vi "Pre Launch Init.vi"(11 "MiniGUI in":refnum<class "MiniGUI.lvclass">) -> (0 "error out":errorcluster, 3 "MiniGUI out":refnum<class "MiniGUI.lvclass">)   [LabVIEW 2019, in "MiniGUI.lvlib" / "MiniGUI.lvclass"]
doc: "Initializes the panel actor. Creates the Panel Helper.\n\n----\nPlease see the following web address for additional documentation and tutorial information:\nhttp://www.mooregoodideas.com/mgi-panel-manager/\n\nAuthor: Derek Trepanier\n\nCopyright (c) 2018, Moore Good Ideas, Inc.\n\nAll rights reserved.\n\nRedistribution and use in source and binary forms, with or without modification, are permitted provided that the following conditions are met:\n\n * Redistributions of source code must retain the above copyright notice, this list of conditions and the following disclaimer.\n * Redistributions in binary form must reproduce the above copyright notice, this list of conditions and the following disclaimer in the documentation and/or other materials provided with the distribution.\n * Neither the name of Moore Good Ideas, Inc. nor the names of its contributors may be used to endorse or promote products derived from this software without specific prior written permission.\n\nTHIS SOFTWARE IS PROVIDED BY THE COPYRIGHT HOLDERS AND CONTRIBUTORS \"AS IS\" AND ANY EXPRESS OR IMPLIED WARRANTIES, INCLUDING, BUT NOT LIMITED TO, THE IMPLIED WARRANTIES OF MERCHANTABILITY AND FITNESS FOR A PARTICULAR PURPOSE ARE DISCLAIMED. IN NO EVENT SHALL THE COPYRIGHT OWNER OR CONTRIBUTORS BE LIABLE FOR ANY DIRECT, INDIRECT, INCIDENTAL, SPECIAL, EXEMPLARY, OR CONSEQUENTIAL DAMAGES (INCLUDING, BUT NOT LIMITED TO, PROCUREMENT OF SUBSTITUTE GOODS OR SERVICES; LOSS OF USE, DATA, OR PROFITS; OR BUSINESS INTERRUPTION) HOWEVER CAUSED AND ON ANY THEORY OF LIABILITY, WHETHER IN CONTRACT, STRICT LIABILITY, OR TORT (INCLUDING NEGLIGENCE OR OTHERWISE) ARISING IN ANY WAY OUT OF THE USE OF THIS SOFTWARE, EVEN IF ADVISED OF THE POSSIBILITY OF SUCH DAMAGE."
uses:
  MiniGUI.lvclass
  Dataset GUI.ctl
  LabGUI Head.ctl
  MiniGUI.lvclass/MiniGUI.ctl
  <vilib>/MGI/Panel Manager/Panel Actor/Panel Actor/Panel Actor.lvclass
  MiniGUI.lvlib
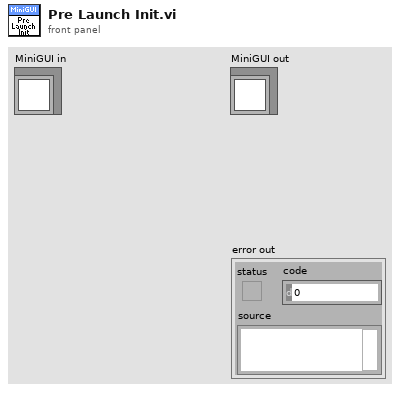
[diagram p1: front panel]
types:
  T1 = typedef "LabGUI Head.ctl" = cluster{"SV":dbl, "PV":dbl, "String":string, "Color Box":u32, "FeedBack":enum16{""}}
  T2 = cluster{"Compressor":bool, "M1":T1, "M2":T1, "Error":string, "System Name":string, "dual head":bool}
  T3 = typedef "MiniGUI.lvlib/Dataset GUI.ctl" = cluster{"M1 Status":cluster{"Read Temp":dbl[unit], "Bin String":string, "M1 Set Temp":dbl[unit], "Feedback":u8}, "M2 Status":cluster{"Read Temp":dbl[unit], "Bin String":string, "M2 Set Temp":dbl[unit], "Feedback":u8}}
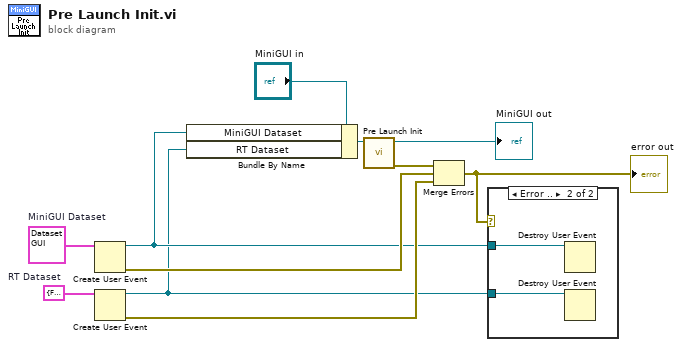
[diagram p0: block diagram]
diagram:
  w2 = T2 {"Compressor"=FALSE, "M1"={"SV"=0.0, "PV"=0.0, "String"="", "Color Box"=0, "FeedBack"=enum.""}, "M2"={"SV"=0.0, "PV"=0.0, "String"="", "Color Box"=0, "FeedBack"=enum.""}, "Error"="", "System Name"="", "dual head"=FALSE}  # RT Dataset
  w4 = T3 {"M1 Status"={"Read Temp"=393.25, "Bin String"="", "M1 Set Temp"=393.65, "Feedback"=1}, "M2 Status"={"Read Temp"=393.25, "Bin String"="", "M2 Set Temp"=393.65, "Feedback"=1}}  # MiniGUI Dataset
  n1 = Create User Event(user event datatype=w4) -> (user event=w3:refnum<user-event>, error out=w7:errorcluster)  [unwired: 1 in]
  n2 = Create User Event(user event datatype=w2) -> (user event=w1:refnum<user-event>, error out=w5:errorcluster)  [unwired: 1 in]
  n3 = Bundle By Name(cluster="MiniGUI in", "MiniGUI Dataset"=w3, "RT Dataset"=w1) -> (w6:refnum<class "MiniGUI.lvclass">)
  n4 = call-parent "Pre Launch Init.vi"("Panel Actor in"=w6) -> ("error out"=w10:errorcluster, "Panel Actor out"=→"MiniGUI out":refnum<class "MiniGUI.lvclass">)  [unwired: 9 in]
  n5 = Merge Errors(w10, w7, w5) -> (w9:errorcluster)
  "error out" <- w9
  n6 = case shown="Error .." w9 {
    tunnel: w3 -> [_ w13]
    tunnel: w1 -> [_ w12]
    frame No Error {
    }
    frame Error {
      n7 = Destroy User Event(user event=w13) -> ()  [unwired: 1 in, 1 out]
      n8 = Destroy User Event(user event=w12) -> ()  [unwired: 1 in, 1 out]
    }
  }
